vi "FireAntsEvent.vi"(8 "error in (no error)":errorcluster, 10 "Rectangle (default: deselect)":T1, 11 "Ants in":refnum<class "Ants.lvclass">) -> (0 "error out":errorcluster, 3 "Ants out":refnum<class "Ants.lvclass">)   [LabVIEW 2021, in "Ants.lvclass"]
uses:
  <resource>/plugins/NIIconEditor/Class/Ants/Ants.lvclass
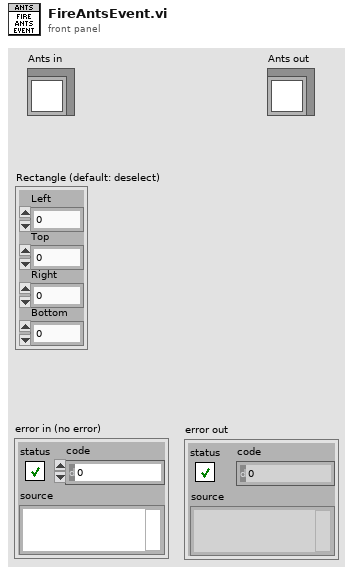
[diagram p1: front panel]
types:
  T1 = cluster{"Left":i32, "Top":i32, "Right":i32, "Bottom":i32}
  T2 = cluster{"Left":i32, "Top":i32, i32, "Bottom":i32}
  T3 = cluster{"Right":i32, "Top":i32, i32, "Bottom":i32}
  T4 = cluster{"Left":i32, "Bottom":i32, "Right":i32, i32}
  T5 = cluster{"Left":i32, "Bottom":i32, "Right":i32, "Bottom":i32}[]
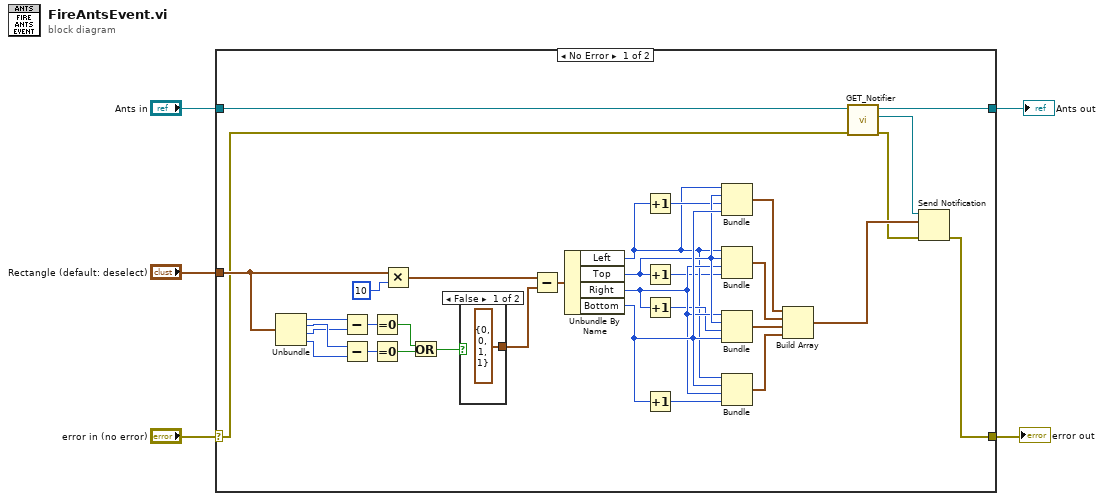
[diagram p0: block diagram]
diagram:
  n1 = case shown="No Error" "error in (no error)" {
    selector: "error in (no error)" -> [w6 w40]
    tunnel: [w11 w41] -> w4
    tunnel: "Ants in" -> [w12 w41]
    tunnel: [w8 w40] -> w2
    tunnel: "Rectangle (default: deselect)" -> [w7 _]
    frame No Error {
      n2 = Unbundle(w7) -> ("Left"=w13:i32, "Top"=w15:i32, "Right"=w14:i32, "Bottom"=w16:i32)
      n3 = Subtract(x=w13, y=w14) -> (x-y=w17:i32)
      n4 = Subtract(x=w15, y=w16) -> (x-y=w18:i32)
      n5 = Equal To 0?(x=w17) -> (x = 0?=w20:bool)
      n6 = Equal To 0?(x=w18) -> (x = 0?=w19:bool)
      n7 = Multiply(x=w7, y=10) -> (x*y=w35:T1)
      n8 = Or(x=w20, y=w19) -> (x .or. y?=w38:bool)
      n9 = case shown="False" w38 {
        tunnel: [T1 {"Left"=0, "Top"=0, "Right"=1, "Bottom"=1} ("y") _] -> w37
        frame False {
        }
        frame True {
        }
      }
      n10 = Subtract(x=w35, y=w37) -> (x-y=w36:T1)
      n11 = Unbundle By Name(w36) -> ("Left"=w23:i32, "Top"=w27:i32, "Right"=w26:i32, "Bottom"=w28:i32)
      n12 = Increment(x=w23) -> (x+1=w24:i32)
      n13 = Increment(x=w27) -> (x+1=w21:i32)
      n14 = Increment(x=w26) -> (x+1=w25:i32)
      n15 = Increment(x=w28) -> (x+1=w22:i32)
      n16 = Bundle("Left"=w23, "Top"=w27, w24, "Bottom"=w28) -> (w32:T2)  [unwired: 1 out]
      n17 = Bundle("Left"=w23, "Top"=w27, "Right"=w26, w21) -> (w31:cluster{"Left":i32, "Top":i32, "Right":i32, i32})  [unwired: 1 out]
      n18 = Bundle("Right"=w26, "Top"=w27, w25, "Bottom"=w28) -> (w30:T3)  [unwired: 1 out]
      n19 = Bundle("Left"=w23, "Bottom"=w28, "Right"=w26, w22) -> (w29:T4)  [unwired: 1 out]
      n20 = Build Array(w32, w31, w30, w29) -> (w33:T5)
      n21 = call-dynamic "GET_Notifier.vi"("error in (no error)"=w6, "Ants.lvclass in"=w12) -> ("error out"=w10:errorcluster, "Notifier"=w9:refnum<notifier>, "Ants.lvclass out"=w11:refnum<class "Ants.lvclass">)  [unwired: 7 out]
      n22 = Send Notification(notification=w33, notifier=w9, error in (no error)=w10) -> (error out=w8:errorcluster)  [unwired: 1 out]
    }
    frame Error {
    }
  }
  "error out" <- w2
  "Ants out" <- w4
